vi "to string 1.0.vi"(8 "error in (no error)":errorcluster, 10 "data in":string, 11 "JSON_RPC_Interface configuration in":refnum<class "JSON_RPC_Interface configuration.lvclass">) -> (0 "error out":errorcluster, 2 "data out":string, 3 "JSON_RPC_Interface configuration out":refnum<class "JSON_RPC_Interface configuration.lvclass">)   [LabVIEW 2018, in "JSON_RPC_Interface configuration.lvclass"]
uses:
  JSON_RPC_Interface configuration.lvclass
  JSON_RPC_Interface configuration.lvclass/JSON_RPC_Interface configuration.ctl
  <vilib>/NI/Tag Bus Module Framework/channel/TBM channel.lvclass
  <vilib>/NI/Configuration Framework/serializable configuration/NISE_CEF_serializable configuration.lvclass
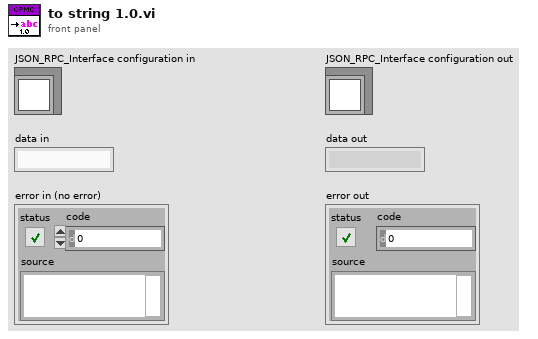
[diagram p1: front panel]
types:
  T1 = typedef "JSON_RPC_Interface configuration.lvclass/Line.ctl" = cluster{"channel":refnum<class "TBM channel.lvclass">}
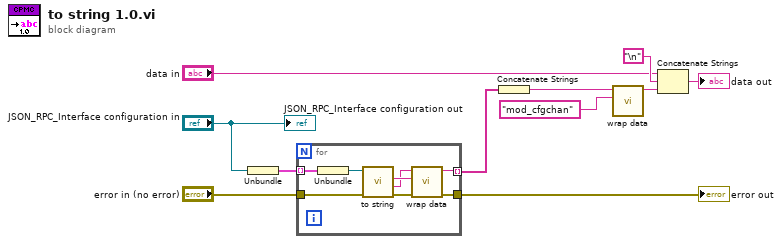
[diagram p0: block diagram]
diagram:
  n1 = Unbundle("JSON_RPC_Interface configuration in") -> (w2:T1[])
  n2 = for {
    tunnel: w2 -> [w18] mode=indexing
    tunnel: [w14] -> w3 mode=indexing
    tunnel: "error in (no error)" -> [w13]
    tunnel: [w12] -> w11
    n3 = Unbundle(w18) -> ("channel"=w17:refnum<class "TBM channel.lvclass">)
    n4 = call-dynamic "to string.vi"("error in"=w13, "channel in"=w17) -> ("error out"=w12:errorcluster, "channel data"=w15:string, "identifier"=w16:string)  [unwired: 6 in, 1 out]
    n5 = call <vilib>:"wrap data.vi"("identifier"=w16, "data to wrap"=w15) -> ("wrapped data"=w14:string)  [unwired: 9 in]
  }
  "error out" <- w11
  n6 = Concatenate Strings(w3) -> (w4:string)
  n7 = call <vilib>:"wrap data.vi"("identifier"="mod_cfgchan", "data to wrap"=w4) -> ("wrapped data"=w8:string)  [unwired: 9 in]
  n8 = Concatenate Strings("data in", "\n", w8) -> (→"data out":string)
  "JSON_RPC_Interface configuration out" <- "JSON_RPC_Interface configuration in"
